vi "LJUD UE9RAW WatchdogRead.vi"(7 "Comm Settings":T1={"Open LabJack "=TRUE, "Use USB"=TRUE, "IP Address"="192.168.1.209", "PortA"=52360, "PortB"=0}, 8 "error in (no error)":errorcluster, 11 "Handle In":i32) -> (0 "error out":errorcluster, 1 "TimeoutPeriod":u16, 2 "WatchdogOptions":u8, 3 "Handle Out":i32, 4 "DAC Parameters":T2, 6 "DIO Parameters":cluster{"DIOConfigA":u8, "DIOConfigB":u8})   [LabVIEW 2021]
panel:
  # "Bit 6:  Reset Comm\nBit 5:  Reset Control\nBit 4:  Update Digital I/O B\nBit 3:  Update Digital I/O A\nBit 1:  Update DAC1 on Timeout\nBit 0:  Update DAC0 on Timeout"
  # "~Seconds"
  # "0-4095"
  # "Bit 7:  State\nBit 4-0:  Digital I/O #"
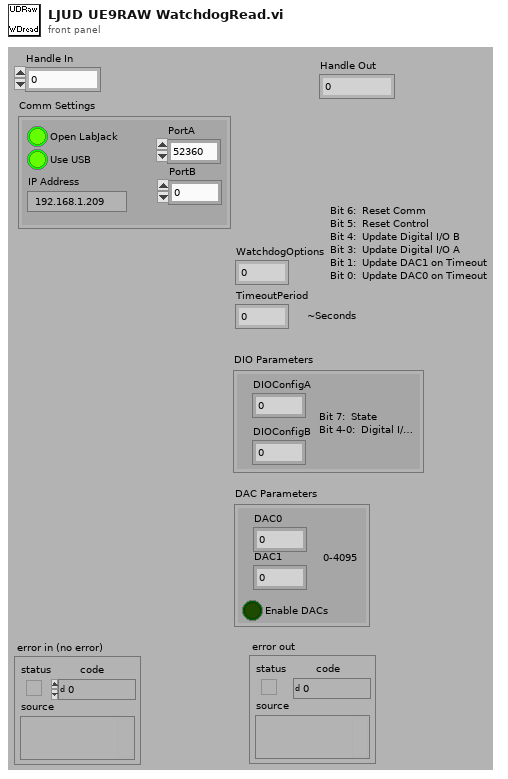
[diagram p1: front panel]
types:
  T1 = cluster{"Open LabJack ":bool, "Use USB":bool, "IP Address":string, "PortA":u16, "PortB":u16}
  T2 = cluster{"DAC0":u16, "DAC1":u16, "Enable DACs":bool}
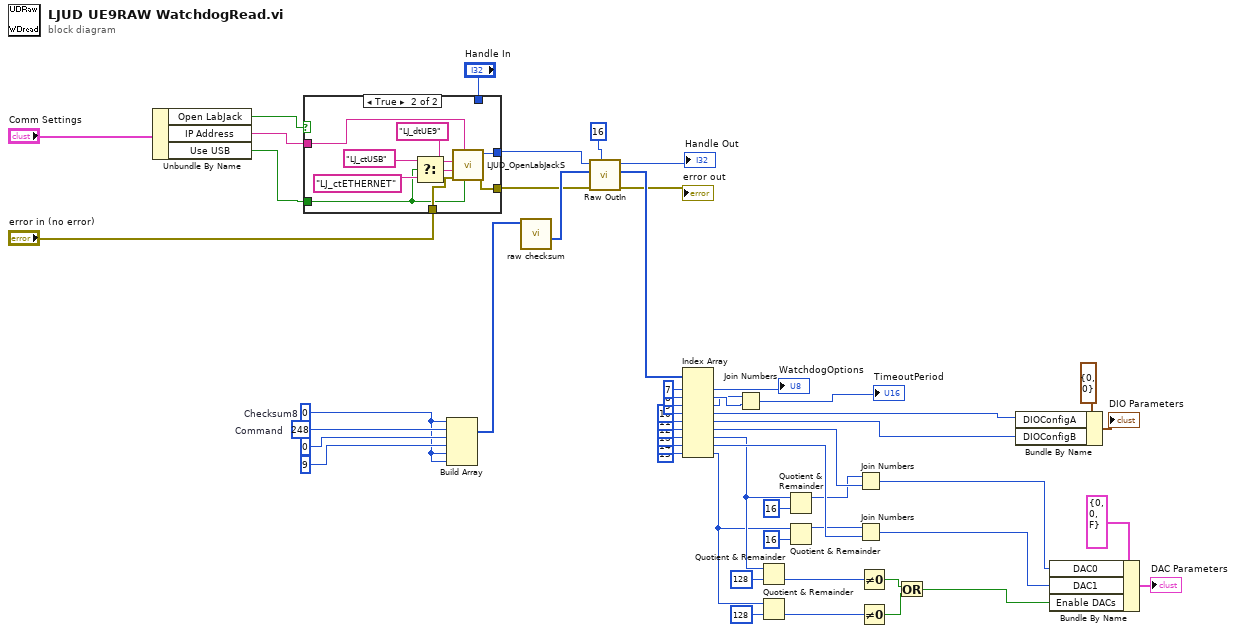
[diagram p0: block diagram]
diagram:
  w51 = u8 0  # Checksum8
  w54 = u8 248  # Command
  n1 = Unbundle By Name("Comm Settings") -> ("Open LabJack"=w12:bool, "IP Address"=w11:string, "Use USB"=w10:bool)
  n2 = case shown="True" w12 {
    tunnel: w11 -> [_ w59]
    tunnel: "error in (no error)" -> [w56 w63]
    tunnel: [w56 w62] -> w9
    tunnel: [w55 w60] -> w8
    tunnel: w10 -> [_ w61]
    tunnel: "Handle In" -> [w55 _]
    frame False {
    }
    frame True {
      n3 = Select(t="LJ_ctUSB" ("ConnectionType"), s=w61, f="LJ_ctETHERNET" ("ConnectionType")) -> (s? t:f=w57:string)
      n4 = call "LJUD_OpenLabJackS.vi"("FirstFound"=w61, "Address"=w59, "error in"=w63, "ConnectionType"=w57, "DeviceType"="LJ_dtUE9") -> ("error out"=w62:errorcluster, "Handle"=w60:i32)  [unwired: 4 in, 1 out]
    }
  }
  n5 = Build Array(w51, w54, u8 0, u8 9, w51, w51) -> (w5:u8[])
  n6 = call "raw checksum.vi"("Array"=w5) -> ("Array Output"=w14:u8[])  [unwired: 3 in, 7 out]
  n7 = call "Raw OutIn.vi"("# of bytes to read in"=16 ("# of bytes to read"), "error in"=w9, "Raw Out"=w14, "Handle In"=w8) -> ("error out"=→"error out":errorcluster, "Raw In"=w4:u8[], "Handle Out"=→"Handle Out":i32)  [unwired: 4 in, 1 out]
  n8 = Index Array(array=w4, index #1=7 ("Index"), index #2=8 ("Index"), index #3=9 ("Index"), index #4=10 ("Index"), index #5=11 ("Index"), index #6=12 ("Index"), index #7=13 ("Index"), index #8=14 ("Index"), index #9=15 ("Index")) -> (element #1=→"WatchdogOptions":u8, element #2=w34:u8, element #3=w33:u8, element #4=w19:u8, element #5=w18:u8, element #6=w31:u8, element #7=w27:u8, element #8=w30:u8, element #9=w26:u8)
  n9 = Join Numbers(hi=w33, lo=w34) -> ((hi.lo)=→"TimeoutPeriod":u16)
  n10 = Quotient & Remainder(x=w27, y=u8 128) -> (floor(x/y)=w38:u8)  [unwired: 1 out]
  n11 = Quotient & Remainder(x=w26, y=u8 128) -> (floor(x/y)=w40:u8)  [unwired: 1 out]
  n12 = Quotient & Remainder(x=w27, y=u8 16) -> (x-y*floor(x/y)=w25:u8)  [unwired: 1 out]
  n13 = Quotient & Remainder(x=w26, y=u8 16) -> (x-y*floor(x/y)=w24:u8)  [unwired: 1 out]
  n14 = Join Numbers(hi=w25, lo=w31) -> ((hi.lo)=w17:u16)
  n15 = Join Numbers(hi=w24, lo=w30) -> ((hi.lo)=w16:u16)
  n16 = Not Equal To 0?(x=w38) -> (x != 0?=w37:bool)
  n17 = Not Equal To 0?(x=w40) -> (x != 0?=w36:bool)
  n18 = Or(x=w37, y=w36) -> (x .or. y?=w15:bool)
  n19 = Bundle By Name(cluster=cluster{"DIOConfigA":u8, "DIOConfigB":u8} {"DIOConfigA"=0, "DIOConfigB"=0} ("DIO Parameters"), "DIOConfigA"=w19, "DIOConfigB"=w18) -> (→"DIO Parameters":cluster{"DIOConfigA":u8, "DIOConfigB":u8})
  n20 = Bundle By Name(cluster=T2 {"DAC0"=0, "DAC1"=0, "Enable DACs"=FALSE} ("DAC Parameters"), "DAC0"=w17, "DAC1"=w16, "Enable DACs"=w15) -> (→"DAC Parameters":T2)
